vi "MemBlock(DBL).vi"(7 "方法":enum16{"初始化", "读取", "读取全部", "写入"}(ring)=enum."读取", 8 "error in (no error)":errorcluster caption="错误输入（无错误）", 9 "索引":i32, 10 "输入值":dbl, 11 "默认值":dbl[](array[numeric])) -> (0 "error out":errorcluster caption="错误输出", 2 "输出值":dbl, 3 "全部数据":dbl[](array[numeric]))   [LabVIEW 2013, in "MemBlock.lvlib"]
uses:
  MemBlock.lvlib
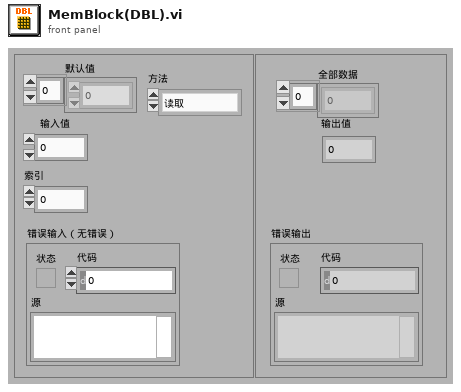
[diagram p1: front panel]
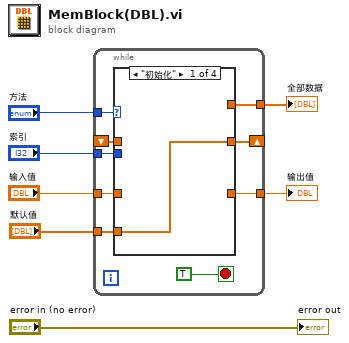
[diagram p0: block diagram]
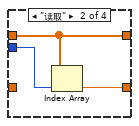
[diagram p2: hidden frame]
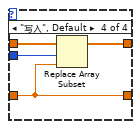
[diagram p4: hidden frame]
diagram:
  n1 = while {
    shift-right: [w14] -> _
    shift-left: _ -> [w13]
    tunnel: "方法" -> [w15]
    tunnel: "输入值" -> [w12]
    tunnel: [w11] -> w5
    tunnel: "索引" -> [w10]
    tunnel: [w9] -> w3
    tunnel: "默认值" -> [w8]
    stop <- TRUE stop-if-true
    n2 = case shown="\"初始化\"" w15 {
      tunnel: [w17 w20 w21 w25] -> w14
      tunnel: w13 -> [_ w20 w21 w23]
      tunnel: w12 -> [_ _ _ w24]
      tunnel: [_ w19 _ w24] -> w11
      tunnel: w10 -> [_ w18 _ w22]
      tunnel: [_ _ w21 _] -> w9
      tunnel: w8 -> [w17 _ _ _]
      frame "初始化" {
      }
      frame "读取" {
        n3 = Index Array(array=w20, index=w18) -> (element=w19:dbl)
      }
      frame "读取全部" {
      }
      frame "写入", Default {
        n4 = Replace Array Subset(array=w23, new element=w24, index=w22) -> (w25:dbl[])
      }
    }
  }
  "输出值" <- w5
  "全部数据" <- w3
  "error out" <- "error in (no error)"
